vi "SubVI_FilterDaqResolutionInfo.vi"(11 "Filtered Command Pairs":u8[][][](array[numeric])=[[[217, 0, 0, 0, 0, 0, 0, 0], [255, 1, 1, 1, 1, 104, 10, 0]]] format="%.0x") -> (2 "MaxOdtEntrySizeDaq":u8, 3 "CmdNotSupported":bool)   [LabVIEW 2019, in "XCP_DaqDtoId.lvlib" / "DAQList.lvclass"]
uses:
  DAQList.lvclass
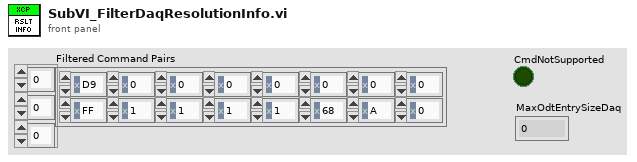
[diagram p1: front panel]
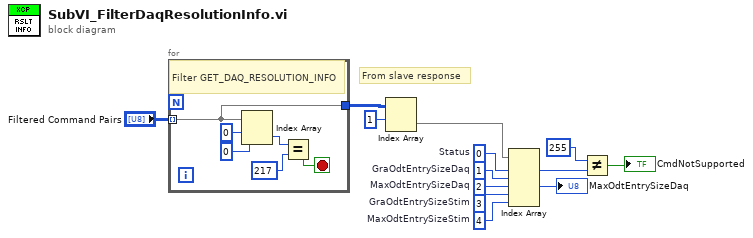
[diagram p0: block diagram]
diagram:
  w1 = 0  # Status
  w6 = 4  # MaxOdtEntrySizeStim
  w7 = 3  # GraOdtEntrySizeStim
  w8 = 2  # MaxOdtEntrySizeDaq
  w9 = 1  # GraOdtEntrySizeDaq
  # "From slave response"
  n1 = for {
    tunnel: "Filtered Command Pairs" -> [w15] mode=indexing
    tunnel: [w15] -> w12
    stop <- w14 stop-if-true
    # "Filter GET_DAQ_RESOLUTION_INFO"
    n2 = Index Array(array=w15, index (row)=0, index (col)=0 ("disabled index (col)")) -> (element=w17:u8)
    n3 = Equal?(x=w17, y=u8 217 ("element")) -> (x = y?=w14:bool)
  }
  n4 = Index Array(array=w12, index (row)=1) -> (element=w10:u8[])  [unwired: 1 in]
  n5 = Index Array(array=w10, index #1=w1, index #2=w9, index #3=w8, index #4=w7, index #5=w6) -> (element #1=w3:u8, element #3=→"MaxOdtEntrySizeDaq":u8)  [unwired: 3 out]
  n6 = Not Equal?(x=u8 255, y=w3) -> (x != y?=→"CmdNotSupported":bool)
